vi "HXG2_Grapher-Scales.vi"(0 "Graph Scales In":dbl[](array[numeric]), 5 "Update Chart":bool, 9 "Scale Ctrl":u32[](array[numeric]), 11 "error in (no error)":errorcluster, 12 "Waveform Chart Ref in":refnum<vi>) -> (15 "error out":errorcluster)   [LabVIEW 2012]
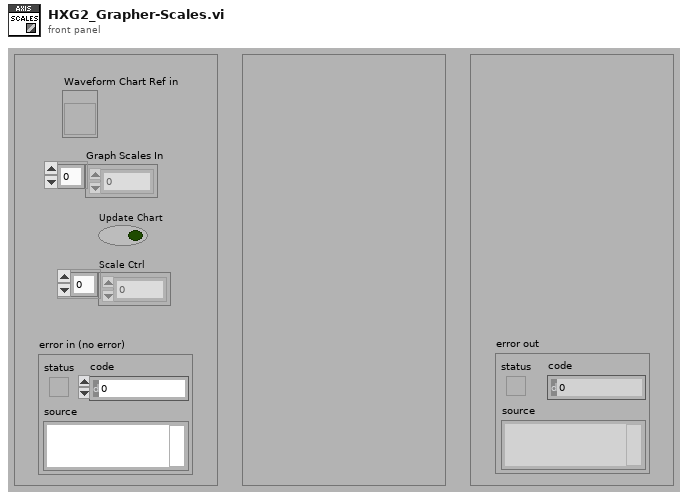
[diagram p1: front panel]
types:
  T1 = cluster{"Graph Scales In[0]":dbl, "Graph Scales In[1]":dbl, "Graph Scales In[2]":dbl, "Graph Scales In[3]":dbl, "Graph Scales In[4]":dbl, "Graph Scales In[5]":dbl, "Graph Scales In[6]":dbl}
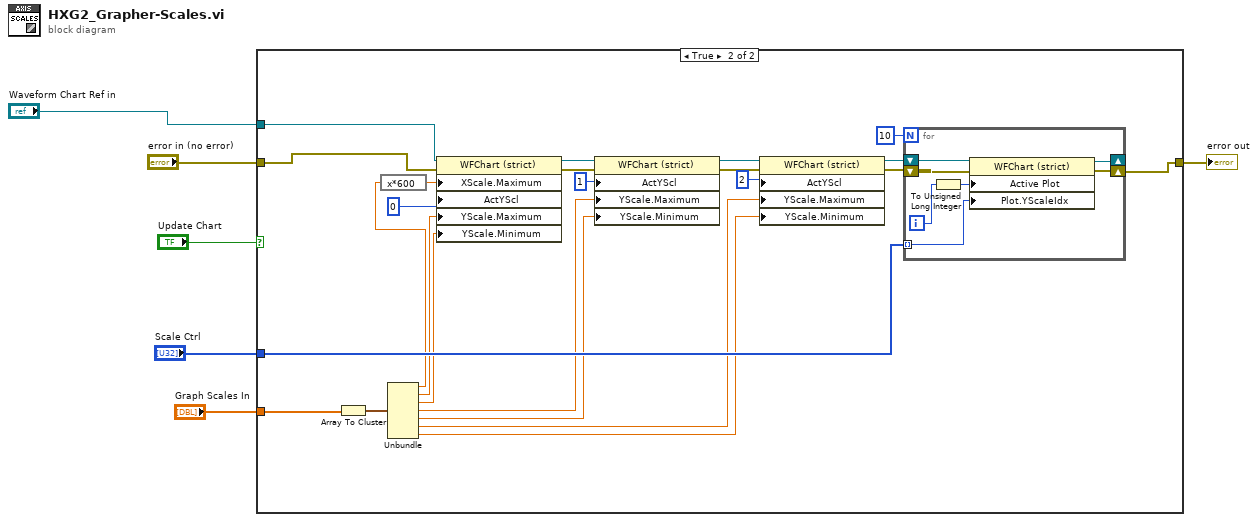
[diagram p0: block diagram]
diagram:
  n1 = case shown="True" "Update Chart" {
    tunnel: "Scale Ctrl" -> [_ w28]
    tunnel: "Waveform Chart Ref in" -> [_ w27]
    tunnel: [w7 w20] -> w3
    tunnel: "error in (no error)" -> [w7 w19]
    tunnel: "Graph Scales In" -> [_ w9]
    frame False {
    }
    frame True {
      n2 = Array To Cluster(array=w9) -> (cluster=w18:T1)
      n3 = Unbundle(w18) -> ("Graph Scales In[0]"=w16:dbl, "Graph Scales In[1]"=w15:dbl, "Graph Scales In[2]"=w14:dbl, "Graph Scales In[3]"=w13:dbl, "Graph Scales In[4]"=w12:dbl, "Graph Scales In[5]"=w11:dbl, "Graph Scales In[6]"=w10:dbl)
      n4 = expression code="x*600"(w16) -> (w31:dbl)
      n5 = property on="Property Node" class="WFChart (strict)"(reference=w27, error in=w19, "XScale.Maximum"=w31, "ActYScl"=0 ("Active Y Scale"), "YScale.Maximum"=w15, "YScale.Minimum"=w14) -> (reference out=w26:refnum<vi>, error out=w25:errorcluster)
      n6 = property on="Property Node" class="WFChart (strict)"(reference=w26, error in=w25, "ActYScl"=1 ("Active Y Scale"), "YScale.Maximum"=w13, "YScale.Minimum"=w12) -> (reference out=w24:refnum<vi>, error out=w23:errorcluster)
      n7 = property on="Property Node" class="WFChart (strict)"(reference=w24, error in=w23, "ActYScl"=2 ("Active Y Scale"), "YScale.Maximum"=w11, "YScale.Minimum"=w10) -> (reference out=w22:refnum<vi>, error out=w21:errorcluster)
      n8 = for {
        N: 10 -> [_]
        tunnel: w28 -> [w34] mode=indexing
        shift-right: [w33] -> w20
        shift-left: w21 -> [w32]
        shift-right: [w37] -> _
        shift-left: w22 -> [w38]
        i -> [w36]
        n9 = To Unsigned Long Integer(number=w36) -> (unsigned 32bit integer=w35:u32)
        n10 = property class="WFChart (strict)"(reference=w38, error in=w32, "Active Plot"=w35, "Plot.YScaleIdx"=w34) -> (reference out=w37:refnum<vi>, error out=w33:errorcluster)
      }
    }
  }
  "error out" <- w3
